vi "公式写入.vi"(7 "公式":cluster{"X^2":dbl, "X":dbl, "b":dbl}, 8 "Error in":errorcluster caption="Error in (no error)", 9 "量程选择":enum16{"低量程", "高量程", "0-2量程"}(ring), 10 "测量模式(公式)":u16(ring)=1 items=["水样测试"=1, "标样核查"=2, "零点核查"=3, "跨度核查"=4, "空白测试"=5, "平行样"=6, "加标回收"=7], 11 "模型":enum32{"线性", "多项式"}(ring)) -> (0 "error out":errorcluster)   [LabVIEW 2016]
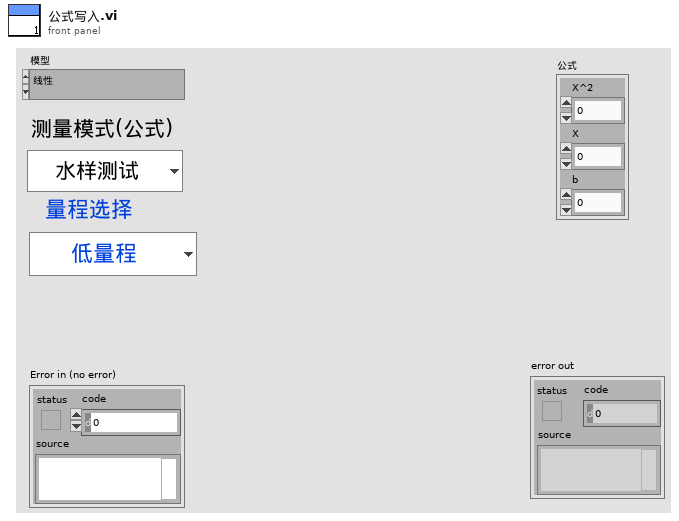
[diagram p1: front panel]
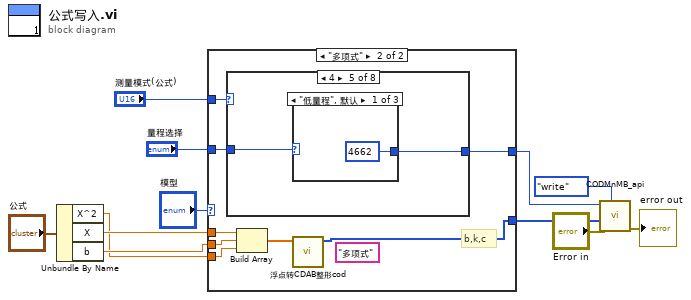
[diagram p0: block diagram]
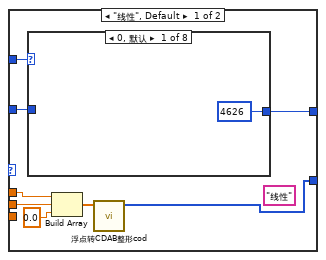
[diagram p2: hidden frame]
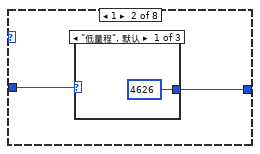
[diagram p3: hidden frame]
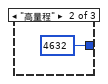
[diagram p4: hidden frame]
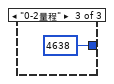
[diagram p5: hidden frame]
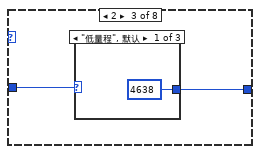
[diagram p6: hidden frame]
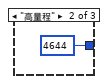
[diagram p7: hidden frame]
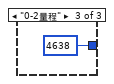
[diagram p8: hidden frame]
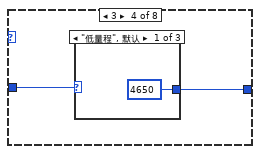
[diagram p9: hidden frame]
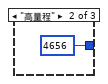
[diagram p10: hidden frame]
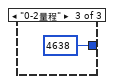
[diagram p11: hidden frame]
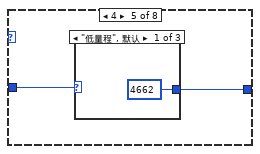
[diagram p12: hidden frame]
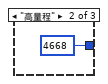
[diagram p13: hidden frame]
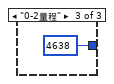
[diagram p14: hidden frame]
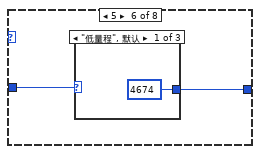
[diagram p15: hidden frame]
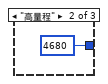
[diagram p16: hidden frame]
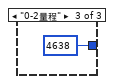
[diagram p17: hidden frame]
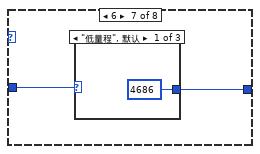
[diagram p18: hidden frame]
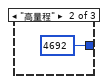
[diagram p19: hidden frame]
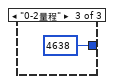
[diagram p20: hidden frame]
diagram:
  n1 = Unbundle By Name("公式") -> ("X^2"=w6:dbl, "X"=w7:dbl, "b"=w8:dbl)
  n2 = case shown="\"多项式\"" "模型" {
    tunnel: [w19 w63] -> w5
    tunnel: [w18 w62] -> w9
    tunnel: w8 -> [w16 w59]
    tunnel: w7 -> [w17 w60]
    tunnel: w6 -> [_ w61]
    tunnel: "测量模式(公式)" -> [w14 w58]
    tunnel: "量程选择" -> [w13 w57]
    frame "线性", Default {
      (unwired) "线性" ("table输入")
      n3 = case shown="0, 默认" w14 {
        tunnel: [u16 4626 ("starting address") w23 w28 w33 w38 w43 w48 w53] -> w19
        tunnel: w13 -> [_ w22 w27 w32 w37 w42 w47 w52]
        frame 0, Default {
        }
        frame 1 {
          n4 = case shown="\"低量程\", 默认" w22 {
            tunnel: [u16 4626 ("starting address") u16 4632 ("starting address") u16 4638 ("starting address")] -> w23
            frame "低量程", Default {
            }
            frame "高量程" {
            }
            frame "0-2量程" {
            }
          }
        }
        frame 2 {
          n5 = case shown="\"低量程\", 默认" w27 {
            tunnel: [u16 4638 ("starting address") u16 4644 ("starting address") u16 4638 ("starting address")] -> w28
            frame "低量程", Default {
            }
            frame "高量程" {
            }
            frame "0-2量程" {
            }
          }
        }
        frame 3 {
          n6 = case shown="\"低量程\", 默认" w32 {
            tunnel: [u16 4650 ("starting address") u16 4656 ("starting address") u16 4638 ("starting address")] -> w33
            frame "低量程", Default {
            }
            frame "高量程" {
            }
            frame "0-2量程" {
            }
          }
        }
        frame 4 {
          n7 = case shown="\"低量程\", 默认" w37 {
            tunnel: [u16 4662 ("starting address") u16 4668 ("starting address") u16 4638 ("starting address")] -> w38
            frame "低量程", Default {
            }
            frame "高量程" {
            }
            frame "0-2量程" {
            }
          }
        }
        frame 5 {
          n8 = case shown="\"低量程\", 默认" w42 {
            tunnel: [u16 4674 ("starting address") u16 4680 ("starting address") u16 4638 ("starting address")] -> w43
            frame "低量程", Default {
            }
            frame "高量程" {
            }
            frame "0-2量程" {
            }
          }
        }
        frame 6 {
          n9 = case shown="\"低量程\", 默认" w47 {
            tunnel: [u16 4686 ("starting address") u16 4692 ("starting address") u16 4638 ("starting address")] -> w48
            frame "低量程", Default {
            }
            frame "高量程" {
            }
            frame "0-2量程" {
            }
          }
        }
        frame 7 {
          n10 = case shown="\"低量程\", 默认" w52 {
            tunnel: [u16 4698 ("starting address") u16 4704 ("starting address") u16 4638 ("starting address")] -> w53
            frame "低量程", Default {
            }
            frame "高量程" {
            }
            frame "0-2量程" {
            }
          }
        }
      }
      n11 = Build Array(w17, w16, 0.0 ("元素")) -> (w20:dbl[])
      n12 = call "浮点转CDAB整形cod.vi"("浮点数"=w20) -> ("CDAB整形输出"=w18:u16[])  [unwired: 10 in]
    }
    frame "多项式" {
      (unwired) "多项式" ("table输入")
      # "b,k,c"
      n13 = case shown="4" w58 {
        tunnel: [u16 4626 ("starting address") w67 w72 w77 w82 w87 w92 w97] -> w63
        tunnel: w57 -> [_ w66 w71 w76 w81 w86 w91 w96]
        frame 0, Default {
        }
        frame 1 {
          n14 = case shown="\"低量程\", 默认" w66 {
            tunnel: [u16 4626 ("starting address") u16 4632 ("starting address") u16 4638 ("starting address")] -> w67
            frame "低量程", Default {
            }
            frame "高量程" {
            }
            frame "0-2量程" {
            }
          }
        }
        frame 2 {
          n15 = case shown="\"低量程\", 默认" w71 {
            tunnel: [u16 4638 ("starting address") u16 4644 ("starting address") u16 4638 ("starting address")] -> w72
            frame "低量程", Default {
            }
            frame "高量程" {
            }
            frame "0-2量程" {
            }
          }
        }
        frame 3 {
          n16 = case shown="\"低量程\", 默认" w76 {
            tunnel: [u16 4650 ("starting address") u16 4656 ("starting address") u16 4638 ("starting address")] -> w77
            frame "低量程", Default {
            }
            frame "高量程" {
            }
            frame "0-2量程" {
            }
          }
        }
        frame 4 {
          n17 = case shown="\"低量程\", 默认" w81 {
            tunnel: [u16 4662 ("starting address") u16 4668 ("starting address") u16 4638 ("starting address")] -> w82
            frame "低量程", Default {
            }
            frame "高量程" {
            }
            frame "0-2量程" {
            }
          }
        }
        frame 5 {
          n18 = case shown="\"低量程\", 默认" w86 {
            tunnel: [u16 4674 ("starting address") u16 4680 ("starting address") u16 4638 ("starting address")] -> w87
            frame "低量程", Default {
            }
            frame "高量程" {
            }
            frame "0-2量程" {
            }
          }
        }
        frame 6 {
          n19 = case shown="\"低量程\", 默认" w91 {
            tunnel: [u16 4686 ("starting address") u16 4692 ("starting address") u16 4638 ("starting address")] -> w92
            frame "低量程", Default {
            }
            frame "高量程" {
            }
            frame "0-2量程" {
            }
          }
        }
        frame 7 {
          n20 = case shown="\"低量程\", 默认" w96 {
            tunnel: [u16 4698 ("starting address") u16 4704 ("starting address") u16 4638 ("starting address")] -> w97
            frame "低量程", Default {
            }
            frame "高量程" {
            }
            frame "0-2量程" {
            }
          }
        }
      }
      n21 = Build Array(w60, w59, w61) -> (w64:dbl[])
      n22 = call "浮点转CDAB整形cod.vi"("浮点数"=w64) -> ("CDAB整形输出"=w62:u16[])  [unwired: 10 in]
    }
  }
  n23 = call "CODMnMB_api.vi"("STEP"=enum16{"open", "read", "write", "close"}."write", "Error in"="Error in", "values"=w9, "starting address"=w5) -> ("error out"=→"error out":errorcluster)  [unwired: 5 in, 2 out]
